vi "AssertConnectorPanesMatchTemplateFiles.vi"(8 "error in (no error)":errorcluster, 9 "absolute custom device xml file":path, 10 "Array":T1(array[cluster]), 11 "TestCase in":refnum<class "TestCase.lvclass">) -> (0 "error out":errorcluster, 3 "TestCase out":refnum<class "TestCase.lvclass">)   [LabVIEW 2027, in "VeriStandTestUtilities.lvlib"]
uses:
  VeriStandTestUtilities.lvlib
  <vilib>/addons/_JKI Toolkits/VI Tester/TestCase.llb/TestCase.lvclass
  <userlib>/_OpenG.lib/array/array.llb/Remove Duplicates from 1D Array (Variant)__ogtk.vi
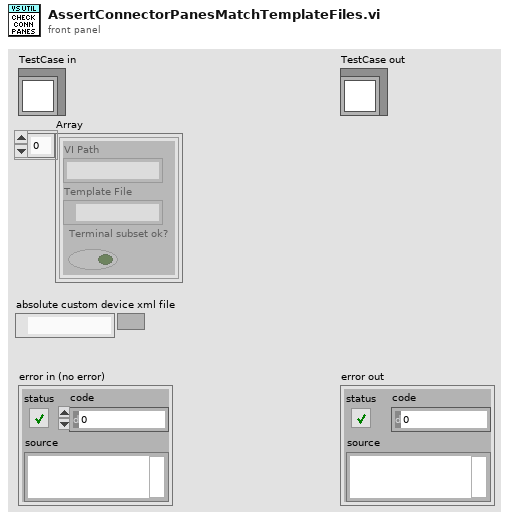
[diagram p1: front panel]
types:
  T1 = cluster{"VI Path":string, "Template File":path, "Terminal subset ok?":bool}[]
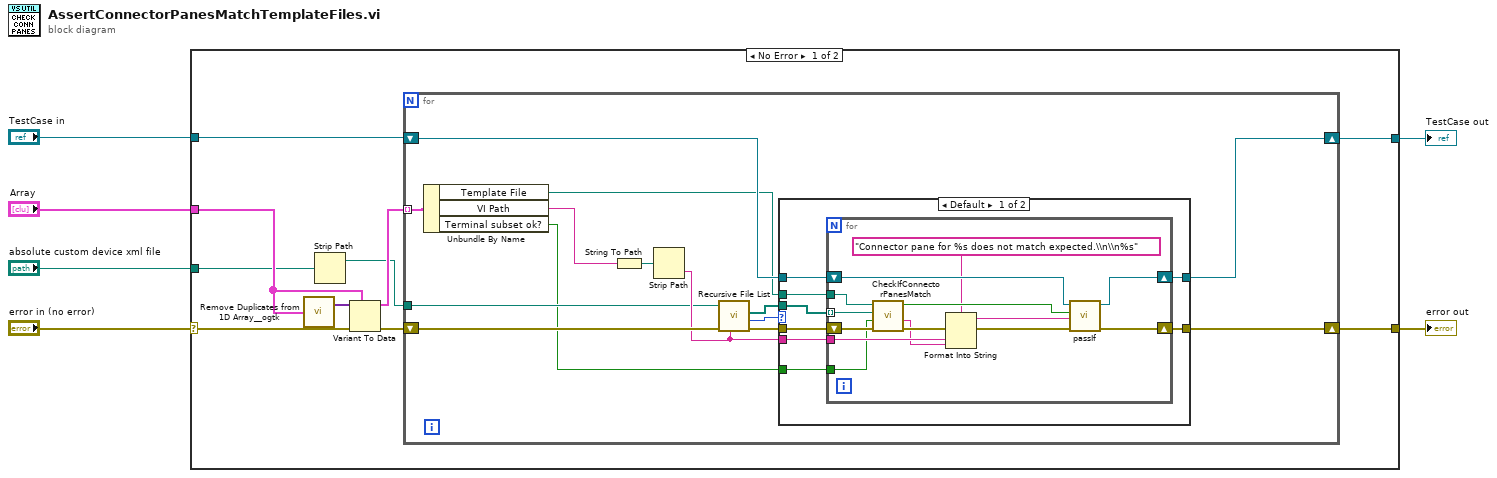
[diagram p0: block diagram]
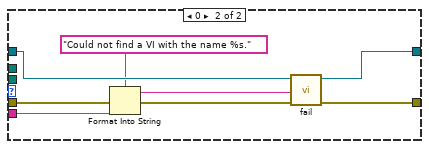
[diagram p2: hidden frame]
diagram:
  n1 = case shown="No Error" "error in (no error)" {
    selector: "error in (no error)" -> [w10 w62]
    tunnel: "absolute custom device xml file" -> [w8 _]
    tunnel: [w16 w61] -> w5
    tunnel: "TestCase in" -> [w15 w61]
    tunnel: [w11 w62] -> w3
    tunnel: "Array" -> [w13 _]
    frame No Error {
      n2 = call-poly <userlib>:"Remove Duplicates from 1D Array__ogtk.vi"("Input Array"=w13) -> ("Output Array"=w14:variant[])  [unwired: 1 out]
      n3 = Strip Path(path=w8) -> (stripped path=w7:path)  [unwired: 1 out]
      n4 = Variant To Data(error in=w10, type=w13, Variant=w14) -> (data=w12:T1, error out=w9:errorcluster)
      n5 = for {
        shift-right: [w28] -> w11
        shift-left: w9 -> [w24]
        tunnel: w12 -> [w27] mode=indexing
        shift-right: [w30] -> w16
        shift-left: w15 -> [w29]
        tunnel: w7 -> [w22]
        n6 = Unbundle By Name(w27) -> ("Template File"=w18:path, "VI Path"=w25:string, "Terminal subset ok?"=w17:bool)
        n7 = String To Path(string=w25) -> (path=w26:path)
        n8 = Strip Path(path=w26) -> (name=w23:string)  [unwired: 1 out]
        n9 = call <vilib>:"Recursive File List.vi"("pattern"=w23, "error in (no error)"=w24, "Folder Path"=w22) -> ("error out"=w20:errorcluster, "Number of Files"=w21:i32, "All Files in Dir"=w19:path[])  [unwired: 4 in, 2 out]
        n10 = case shown="Default" w21 {
          tunnel: w20 -> [w38 w56]
          tunnel: [w36 w60] -> w28
          tunnel: w19 -> [w33 _]
          tunnel: w18 -> [w37 _]
          tunnel: w29 -> [w35 w59]
          tunnel: [w34 w58] -> w30
          tunnel: w23 -> [w32 w57]
          tunnel: w17 -> [w31 _]
          frame Default {
            n11 = for {
              tunnel: w37 -> [w51]
              shift-right: [w49] -> w36
              shift-left: w38 -> [w52]
              shift-right: [w47] -> w34
              shift-left: w35 -> [w48]
              tunnel: w33 -> [w46] mode=indexing
              tunnel: w32 -> [w44]
              tunnel: w31 -> [w39]
              n12 = call "CheckIfConnectorPanesMatch.vi"("error in (no error)"=w52, "terminal subset acceptable (false)"=w39, "actual connector pane vi"=w46, "expected connector pane vi"=w51) -> ("error out"=w42:errorcluster, "mismatch explanation"=w40:string, "connector panes match"=w50:bool)  [unwired: 5 in]
              n13 = Format Into String(format string="Connector pane for %s does not match expected.\\n\\n%s" ("connector pane mismatch error"), error in=w42, w44, w40) -> (resulting string=w43:string, error out=w45:errorcluster)  [unwired: 1 in]
              n14 = call-dynamic "passIf.vi"("error in (no error)"=w45, "message (\"\")"=w43, "pass"=w50, "TestCase in"=w48) -> ("error out"=w49:errorcluster, "TestCase out"=w47:refnum<class "TestCase.lvclass">)  [unwired: 6 in]
            }
          }
          frame 0 {
            n15 = Format Into String(format string="Could not find a VI with the name %s." ("no matches error"), error in=w56, w57) -> (resulting string=w54:string, error out=w55:errorcluster)  [unwired: 1 in]
            n16 = call-dynamic "fail.vi"("error in (no error)"=w55, "message (\"\")"=w54, "TestCase in"=w59) -> ("error out"=w60:errorcluster, "TestCase out"=w58:refnum<class "TestCase.lvclass">)  [unwired: 7 in]
          }
        }
      }
    }
    frame Error {
    }
  }
  "TestCase out" <- w5
  "error out" <- w3
